vi "Create Facade (byURL).vi"(5 "SMOFacade in":refnum<class "SMOFacade.lvclass">, 6 "Filters":string[](array[string]), 8 "error in (no error)":errorcluster, 11 "URL":string) -> (0 "error out":errorcluster, 3 "SMOFacade out":refnum<class "SMOFacade.lvclass">)   [LabVIEW 2021, in "smo.lvlib" / "SMOFacade.lvclass"]
uses:
  SMOFacade.lvclass
  SMOFacade.lvclass/SMOFacade.ctl
  <vilib>/Utility/error.llb/Error Cluster From Error Code.vi
  <vilib>/ErrorRing/Error Ring.xnode
  Registry/Registry-SMO.lvclass
  URI Parsing/URI.lvlib
  SMO/SMO.lvclass
  PublicEvents/PublicEvents.lvclass
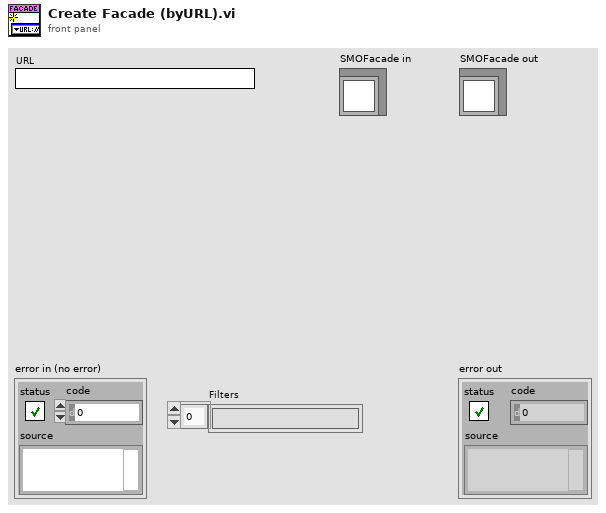
[diagram p1: front panel]
types:
  T1 = typedef "smo.lvlib/Registry-SMO.lvclass/SMO_API--Cluster.ctl" = cluster{"Method Name":string, "Full Method Name":string, "SMO Input":refnum<class "Terminal.lvclass">, "SMO Output":refnum<class "Terminal.lvclass">, "Inputs":refnum<class "Terminal.lvclass">[], "Outputs":refnum<class "Terminal.lvclass">[], "Error Output":refnum<class "Terminal.lvclass">, "vi reference":refnum<vi>}
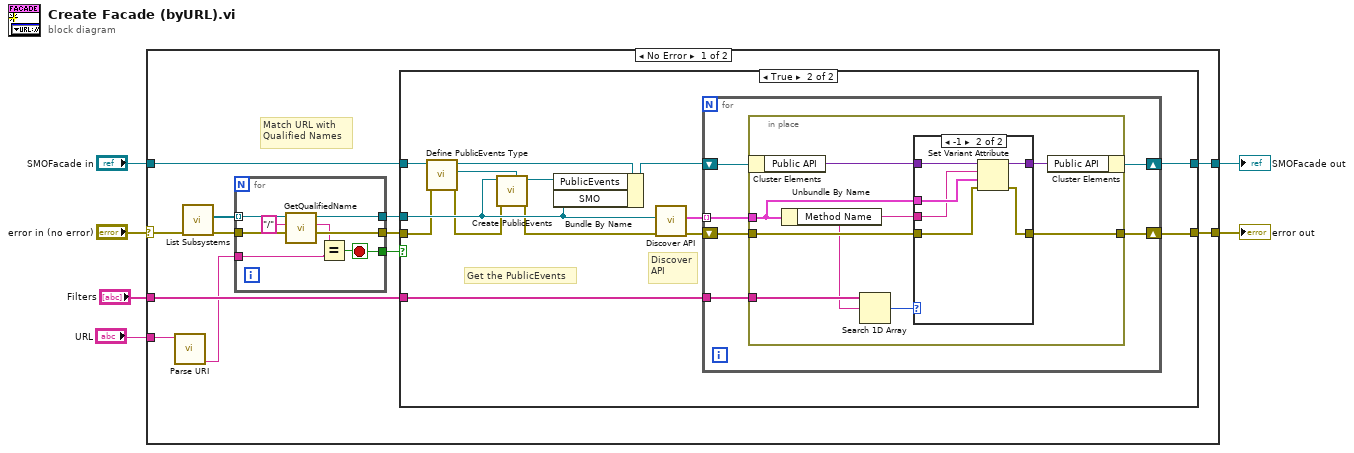
[diagram p0: block diagram]
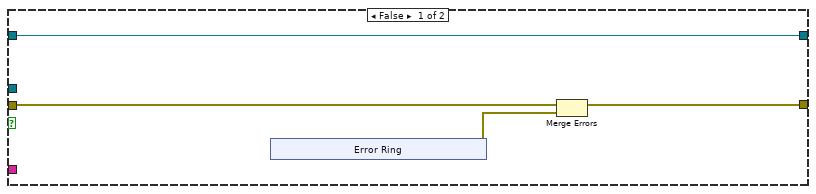
[diagram p2: hidden frame]
diagram:
  n1 = case shown="No Error" "error in (no error)" {
    selector: "error in (no error)" -> [w14 w72]
    tunnel: [w16 w72] -> w5
    tunnel: [w17 w71] -> w3
    tunnel: "SMOFacade in" -> [w18 w71]
    tunnel: "URL" -> [w13 _]
    tunnel: "Filters" -> [w15 _]
    frame No Error {
      # "Match URL with\nQualified Names"
      n2 = call "Parse URI.vi"("URI"=w13) -> ("path"=w9:string)  [unwired: 6 in, 4 out]
      n3 = call "List Subsystems.vi"("error in (no error)"=w14) -> ("error out"=w11:errorcluster, "Subsystems"=w12:refnum<class "SMO.lvclass">[])  [unwired: 9 in]
      n4 = for {
        tunnel: w12 -> [w70] mode=indexing
        tunnel: w9 -> [w67]
        tunnel: [w65] -> w8
        tunnel: [w64] -> w7
        tunnel: w11 -> [w69]
        tunnel: [w68] -> w10
        stop <- w64 stop-if-true
        n5 = call "GetQualifiedName.vi"("error in (no error)"=w69, "separator (dot)"="/", "SMO"=w70) -> ("error out"=w68:errorcluster, "Qualified Name"=w66:string, "SMO out"=w65:refnum<class "SMO.lvclass">)  [unwired: 6 in]
        n6 = Equal?(x=w66, y=w67) -> (x = y?=w64:bool)
      }
      n7 = case shown="True" w7 {
        tunnel: w18 -> [w22 w31]
        tunnel: [w22 w39] -> w17
        tunnel: [w19 w36] -> w16
        tunnel: w15 -> [_ w35]
        tunnel: w10 -> [w21 w28]
        tunnel: w8 -> [_ w33]
        frame False {
          n8 = xnode "Error Ring"() -> ("error out"=w20:errorcluster)
          n9 = Merge Errors(w21, w20) -> (w19:errorcluster)
        }
        frame True {
          # "Discover\nAPI"
          # "Get the PublicEvents"
          n10 = call-dynamic "Define PublicEvents Type.vi"("error in (no error)"=w28, "SMOFacade in"=w31) -> ("error out"=w27:errorcluster, "PublicEvents type"=w29:refnum<class "PublicEvents.lvclass">, "SMOFacade out"=w30:refnum<class "SMOFacade.lvclass">)  [unwired: 7 in]
          n11 = call "Create PublicEvents.vi"("PublicEvents in"=w29, "error in (no error)"=w27, "SMO"=w33) -> ("error out"=w32:errorcluster, "PublicEvents"=w34:refnum<class "PublicEvents.lvclass">)  [unwired: 7 in]
          n12 = Bundle By Name(cluster=w30, "PublicEvents"=w34, "SMO"=w33) -> (w40:refnum<class "SMOFacade.lvclass">)
          n13 = call "Discover API.vi"("error in (no error)"=w32, "SMO"=w33) -> ("error out"=w37:errorcluster, "PublicAPI"=w38:T1[])  [unwired: 8 in]
          n14 = for {
            shift-right: [w45] -> w39
            shift-left: w40 -> [w46]
            tunnel: w38 -> [w44] mode=indexing
            shift-right: [w42] -> w36
            shift-left: w37 -> [w43]
            tunnel: w35 -> [w41]
            n15 = in-place {
              in-place-border: w44 -> [w53]
              in-place-border: w43 -> [w51]
              in-place-border: [w50] -> w42
              in-place-border: w41 -> [w49]
              n16 = in-place-cluster #1(w46) -> ("Public API"=w54:variant)
              n17 = Unbundle By Name(w53) -> ("Method Name"=w48:string)
              n18 = Search 1D Array(1D array=w49, element=w48) -> (index of element=w47:i32)  [unwired: 1 in]
              n19 = case shown="-1" w47 {
                tunnel: w54 -> [w56 w62]
                tunnel: w53 -> [_ w61]
                tunnel: [w56 w60] -> w52
                tunnel: w51 -> [w55 w59]
                tunnel: [w55 w58] -> w50
                tunnel: w48 -> [_ w57]
                frame Default {
                }
                frame -1 {
                  n20 = Set Variant Attribute(Variant=w62, name=w57, value=w61, error in=w59) -> (Variant out=w60:variant, error out=w58:errorcluster)  [unwired: 1 out]
                }
              }
              n21 = in-place-cluster #1("Public API"=w52) -> (w45:refnum<class "SMOFacade.lvclass">)
            }
          }
        }
      }
    }
    frame Error {
    }
  }
  "error out" <- w5
  "SMOFacade out" <- w3
